vi "DeviceOn.vi"(8 "error in (no error)":errorcluster, 11 "NhRegenGridSim in":refnum<class "NhRegenGridSim.lvclass">) -> (0 "error out":errorcluster, 3 "NhRegenGridSim out":refnum<class "NhRegenGridSim.lvclass">)   [LabVIEW 2018, in "AcPwrPlugins.lvlib" / "NhRegenGridSim.lvclass"]
uses:
  NhRegenGridSim.lvclass
  C:/Users/ico/Documents/Projects/NistPluggableModules/AcPwr/AcPwrPlugins/AcPwrBaseClass/AcPwrBase.lvclass
  AcPwrBaseClass/AcPwrBase.lvclass/AcPwrBase.ctl
  AcPwrBaseClass/Accessors/Read Phases.vi
  <instrlib>/NH Research 9400 Series/NH Research 9400 Series.lvlib
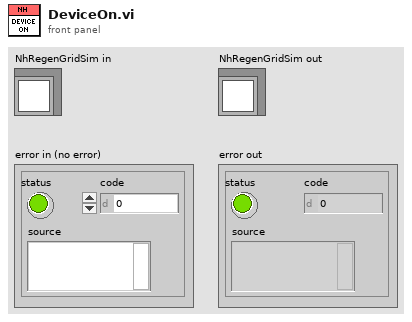
[diagram p1: front panel]
types:
  T1 = typedef "AcPwrPlugins.lvlib/AcPwrBase.lvclass/Phase.ctl" = cluster{"Enabled":bool, "VoltageLevel":dbl, "Waveform":string, "Name":string, "VoltageRange":dbl[], "CurrentLimit":dbl, "Handle":string, "Connected":bool}
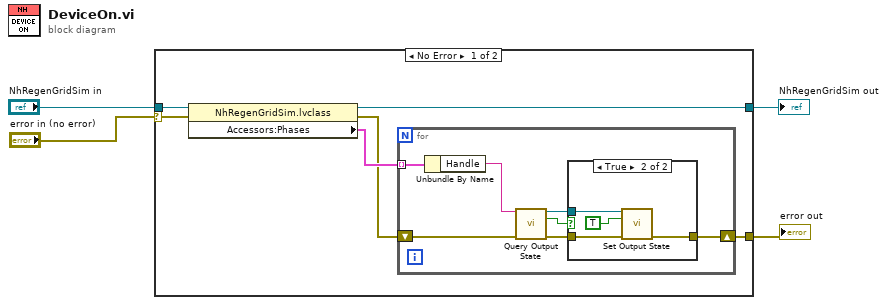
[diagram p0: block diagram]
diagram:
  n1 = case shown="No Error" "error in (no error)" {
    selector: "error in (no error)" -> [w9 w23]
    tunnel: "NhRegenGridSim in" -> [w10 w24]
    tunnel: [w7 w24] -> w2
    tunnel: [w5 w23] -> w1
    frame No Error {
      n2 = property class="NhRegenGridSim.lvclass"(reference=w10, error in=w9) -> (reference out=w7:refnum<class "NhRegenGridSim.lvclass">, error out=w6:errorcluster, "Accessors:Phases"=w8:T1[])
      n3 = for {
        tunnel: w8 -> [w17] mode=indexing
        shift-right: [w13] -> w5
        shift-left: w6 -> [w16]
        n4 = Unbundle By Name(w17) -> ("Handle"=w12:string)
        n5 = call <instrlib>:"Query Output State.vi"("VISA resource name"=w12, "error in (no error)"=w16) -> ("VISA resource name out"=w11:refnum<visa-resource-name>, "Output Enabled"=w15:bool, "error out"=w14:errorcluster)  [unwired: 11 in]
        n6 = case shown="True" w15 {
          tunnel: w14 -> [w18 w22]
          tunnel: [w18 w21] -> w13
          tunnel: w11 -> [_ w20]
          frame False {
          }
          frame True {
            n7 = call <instrlib>:"Set Output State.vi"("VISA resource name"=w20, "Output State (F: Disable)"=TRUE, "error in (no error)"=w22) -> ("error out"=w21:errorcluster)  [unwired: 11 in, 1 out]
          }
        }
      }
    }
    frame Error {
    }
  }
  "error out" <- w1
  "NhRegenGridSim out" <- w2
